vi "Get Configuration File Path.vi"() -> (3 "Configuration File Path":path)   [LabVIEW 2027, in "Embedded Data Logger System Explorer.lvlib"]
uses:
  Embedded Data Logger System Explorer.lvlib
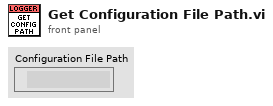
[diagram p1: front panel]
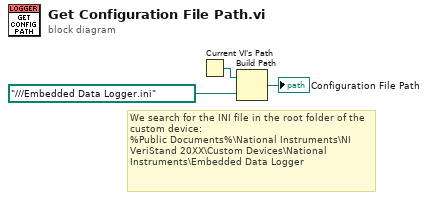
[diagram p0: block diagram]
diagram:
  # "We search for the INI file in the root folder of the custom device:\n%Public Documents%\\National Instruments\\NI VeriStand 20XX\\Custom Devices\\National Instruments\\Embedded Data Logger"
  n1 = Current VI's Path() -> (path=w2:path)
  n2 = Build Path(base path=w2, name or relative path=path "../../../Embedded Data Logger.ini") -> (appended path=→"Configuration File Path":path)
